vi "PFI-28000-Base-Constant_Response Dequeue Timeout.vi"() -> (6 "Timeout":i32)   [LabVIEW 2017, in "PFI-28000-Base.lvclass"]
uses:
  PFI-28000-Base.lvclass
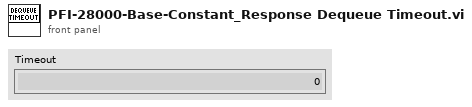
[diagram p1: front panel]
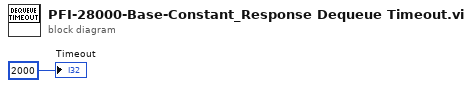
[diagram p0: block diagram]
diagram:
  "Timeout" <- 2000 ("timeout in ms (-1)")
